vi "BubbleSort.vi"(11 "Unsorted Array":T1(array[cluster]) {"End" format="%<%.3X>T"; "Start" format="%<%.3X>T"}) -> (3 "Sorted Array":T1(array[cluster]) {"End" format="%<%.3X>T"; "Start" format="%<%.3X>T"})   [LabVIEW 2017]
panel:
  out "Partially Sorted":T1(array[cluster]) {"End" format="%<%.3X>T"; "Start" format="%<%.3X>T"}
  out "Flipped":bool
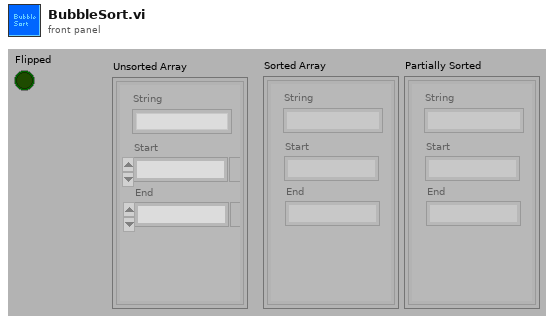
[diagram p1: front panel]
types:
  T1 = cluster{"String":string, "Start":timestamp, "End":timestamp}[]
  T2 = cluster{"String":string, "Start":timestamp, "End":timestamp}
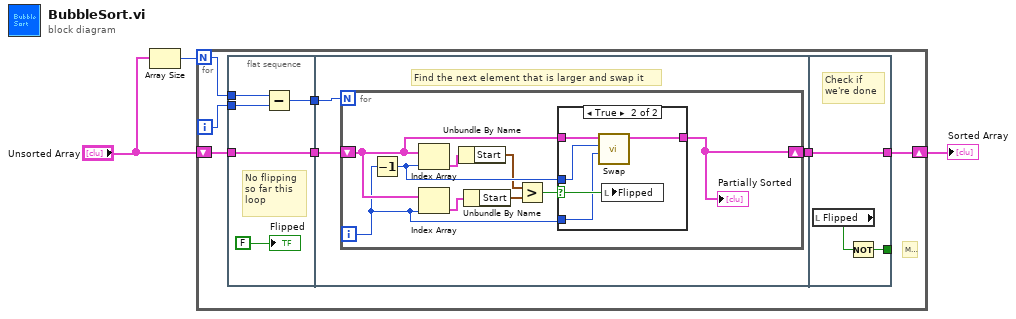
[diagram p0: block diagram]
diagram:
  # "Missing object. The object \"Loop Condition\" does not exist in the previous version."
  n1 = Array Size(array="Unsorted Array") -> (size(s)=w3:i32)
  n2 = for {
    N: w3 -> [w7]
    shift-right: [w9] -> w1
    shift-left: "Unsorted Array" -> [w10]
    i -> [w4]
    n3 = flat-sequence {
      tunnel: w4 -> [w13]
      tunnel: w7 -> [w14]
      tunnel: w10 -> [w15]
      tunnel: [w15] -> w6
      tunnel: [w12] -> w5
      tunnel: [w17] -> w8
      tunnel: w6 -> [w18]
      tunnel: w5 -> [w16]
      tunnel: [w36] -> w9
      tunnel: w8 -> [w36]
      tunnel: [w34] -> _
      frame #0 {
        # "No flipping\nso far this\nloop"
        n4 = Subtract(x=w14, y=w13) -> (x-y=w12:i32)
        "Flipped" <- FALSE ("Flipped")
      }
      frame #1 {
        # "Find the next element that is larger and swap it"
        n5 = for {
          N: w16 -> [_]
          shift-right: [w23] -> w17
          shift-left: w18 -> [w26]
          i -> [w25]
          n6 = Decrement(x=w25) -> (x-1=w24:i32)
          n7 = Index Array(array=w26, index=w24) -> (element=w22:T2)
          n8 = Index Array(array=w26, index=w25) -> (element=w20:T2)
          n9 = Unbundle By Name(w22) -> ("Start"=w21:timestamp)
          n10 = Unbundle By Name(w20) -> ("Start"=w19:timestamp)
          n11 = Greater?(x=w21, y=w19) -> (0:w27:bool)
          n12 = case shown="True" w27 {
            selector: w27 -> [_ w33]
            tunnel: w26 -> [w28 w32]
            tunnel: w24 -> [_ w31]
            tunnel: w25 -> [_ w30]
            tunnel: [w28 w29] -> w23
            frame False {
            }
            frame True {
              n13 = call "Swap.vi"("Y"=w30, "X"=w31, "Unswapped Array"=w32) -> ("Swapped Array"=w29:T1)  [unwired: 8 out]
              n14 = local write "Flipped"(w33) -> ()
            }
          }
          "Partially Sorted" <- w23
        }
      }
      frame #2 {
        # "Check if\nwe're done"
        n15 = local read "Flipped"() -> (w35:bool)
        n16 = Not(x=w35) -> (.not. x?=w34:bool)
      }
    }
  }
  "Sorted Array" <- w1
